vi "Read Stop Iterate Notifier.vi"(8 "error in (no error)":errorcluster, 11 "Abstract Iterator Actor in":refnum<class "Abstract Iterator Actor.lvclass">) -> (0 "error out":errorcluster, 2 "Stop Iterate Notifier":refnum<notifier>, 3 "Abstract Iterator Actor out":refnum<class "Abstract Iterator Actor.lvclass">)   [LabVIEW 2023, in "Iterator Actor.lvlib" / "Abstract Iterator Actor.lvclass"]
uses:
  Abstract Iterator Actor.lvclass
  Abstract Iterator Actor.lvclass/Abstract Iterator Actor.ctl
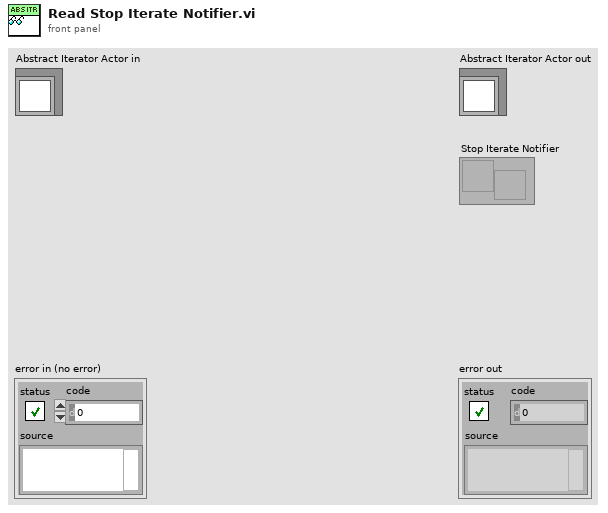
[diagram p1: front panel]
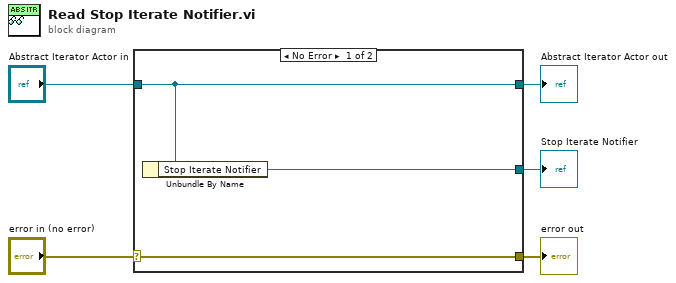
[diagram p0: block diagram]
diagram:
  n1 = case shown="No Error" "error in (no error)" {
    selector: "error in (no error)" -> [w8 w9]
    tunnel: [w8 w9] -> w4
    tunnel: [w7 w10] -> w2
    tunnel: "Abstract Iterator Actor in" -> [w7 w10]
    tunnel: [w6 _] -> w1
    frame No Error {
      n2 = Unbundle By Name(w7) -> ("Stop Iterate Notifier"=w6:refnum<notifier>)
    }
    frame Error {
    }
  }
  "error out" <- w4
  "Abstract Iterator Actor out" <- w2
  "Stop Iterate Notifier" <- w1
